vi "Set RPM.vi"(2 "Gain Vbus":dbl=0.02, 3 "Range RPM":dbl=100.0, 4 "Set Point RPM":dbl, 5 "EncoderDevRef":T1={"DevStatus"={"status"=FALSE, "code"=0, "source"=""}, "EncoderIndex"=enum."Invalid", "CounterIndex"=enum."Ctr 1", "DistancePerCount"=2.0, "Decoding Type"=enum."4x"}) -> (0 "Vbus Out":dbl, 1 "READY!":bool)   [LabVIEW 2012]
uses:
  <vilib>/Rock Robotics/WPI/Encoder/WPI_EncoderDevRef.ctl
  <vilib>/Rock Robotics/SystemInterfaces/Encoder/FPGA_EncoderIdx.ctl
  <vilib>/Rock Robotics/SystemInterfaces/Counter/FPGA_CounterCtrSystemIndex.ctl
  <vilib>/Rock Robotics/WPI/Encoder/WPI_EncoderType.ctl
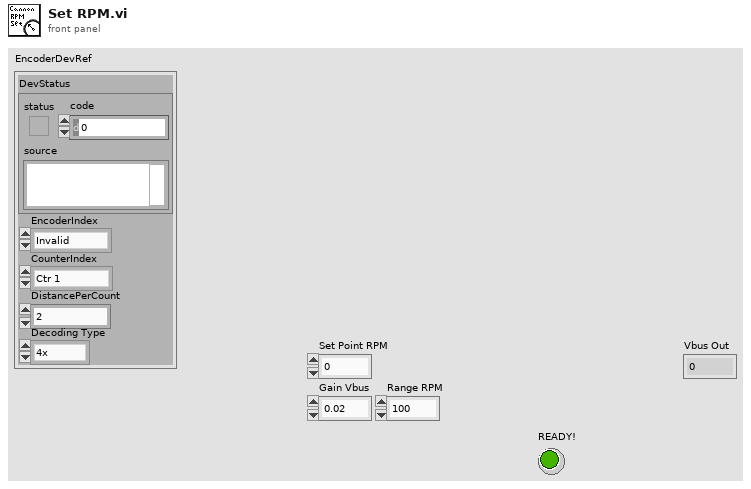
[diagram p1: front panel]
types:
  T1 = typedef "WPI_EncoderDevRef.ctl" = cluster{"DevStatus":errorcluster, "EncoderIndex":T2, "CounterIndex":T3, "DistancePerCount":dbl, "Decoding Type":T4}
  T2 = typedef "FPGA_EncoderIdx.ctl" = enum8{"Enc 0", "Enc 1", "Enc 2", "Enc 3", "Invalid"}
  T3 = typedef "FPGA_CounterCtrSystemIndex.ctl" = enum8{"Ctr 0", "Ctr 1", "Ctr 2", "Ctr 3", "Ctr 4", "Ctr 5", "Ctr 6", "Ctr 7", "Invalid"}
  T4 = typedef "WPI_EncoderType.ctl" = enum16{"1x", "2x", "4x"}
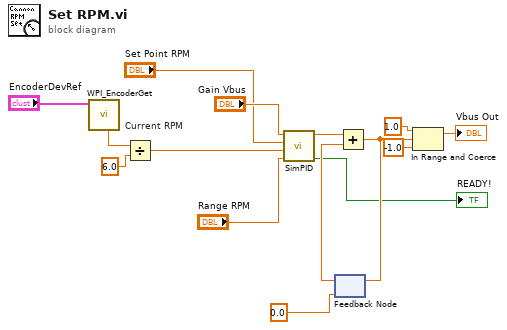
[diagram p0: block diagram]
diagram:
  n1 = call <vilib>:"WPI_EncoderGet.vi"("EncoderDevRef"="EncoderDevRef") -> ("Rate"=w15:dbl)  [unwired: 5 in, 5 out]
  n2 = Divide "Current RPM"(x=w15, y=6.0) -> (x/y=w11:dbl)
  n3 = call "SimPID.vi"("Range"="Range RPM", "Position"=w11, "Set Point"="Set Point RPM", "Gain"="Gain Vbus") -> ("On Target"=→"READY!":bool, "result"=w6:dbl)  [unwired: 5 in]
  n4 = feedback #1(0.0) -> (w10:dbl)
  n5 = Add(x=w6, y=w10) -> (x+y=w9:dbl)
  n6 = feedback-in #1(w9) -> ()
  n7 = In Range and Coerce(upper limit=1.0, x=w9, lower limit=-1.0) -> (coerced(x)=→"Vbus Out":dbl)  [unwired: 1 out]
